vi "eGateHSP_Init.vi"(0 "e.gate Configuration":T1 {"StartTime" format="%#.10f"; "dActTimeToSecondFactor" format="%#.10f"; "StartTimeToDayFactor" format="%#_10f"}, 1 "DLL Path":path, 5 "IP-Adresse":string, 7 "mode":i32, 9 "sampleRate":i32, 11 "error in":errorcluster caption="Fehler (Eingang, kein Fehler)", 12 "timeout":i32) -> (4 "e.gate Configuration 2":T1 {"StartTime" format="%#.10f"; "dActTimeToSecondFactor" format="%#.10f"; "StartTimeToDayFactor" format="%#_10f"}, 15 "Fehler (Ausgang)":errorcluster)   [LabVIEW 2016]
uses:
  e.gate Configuration.ctl
  e.gate Channel Data.ctl
  e.gate Data Type.ctl
  e.gate Protocol Type.ctl
  e.gate Module  Data.ctl
  e.gateHSP_DLLhandle.ctl
panel:
  out "Rückgabewert":i32
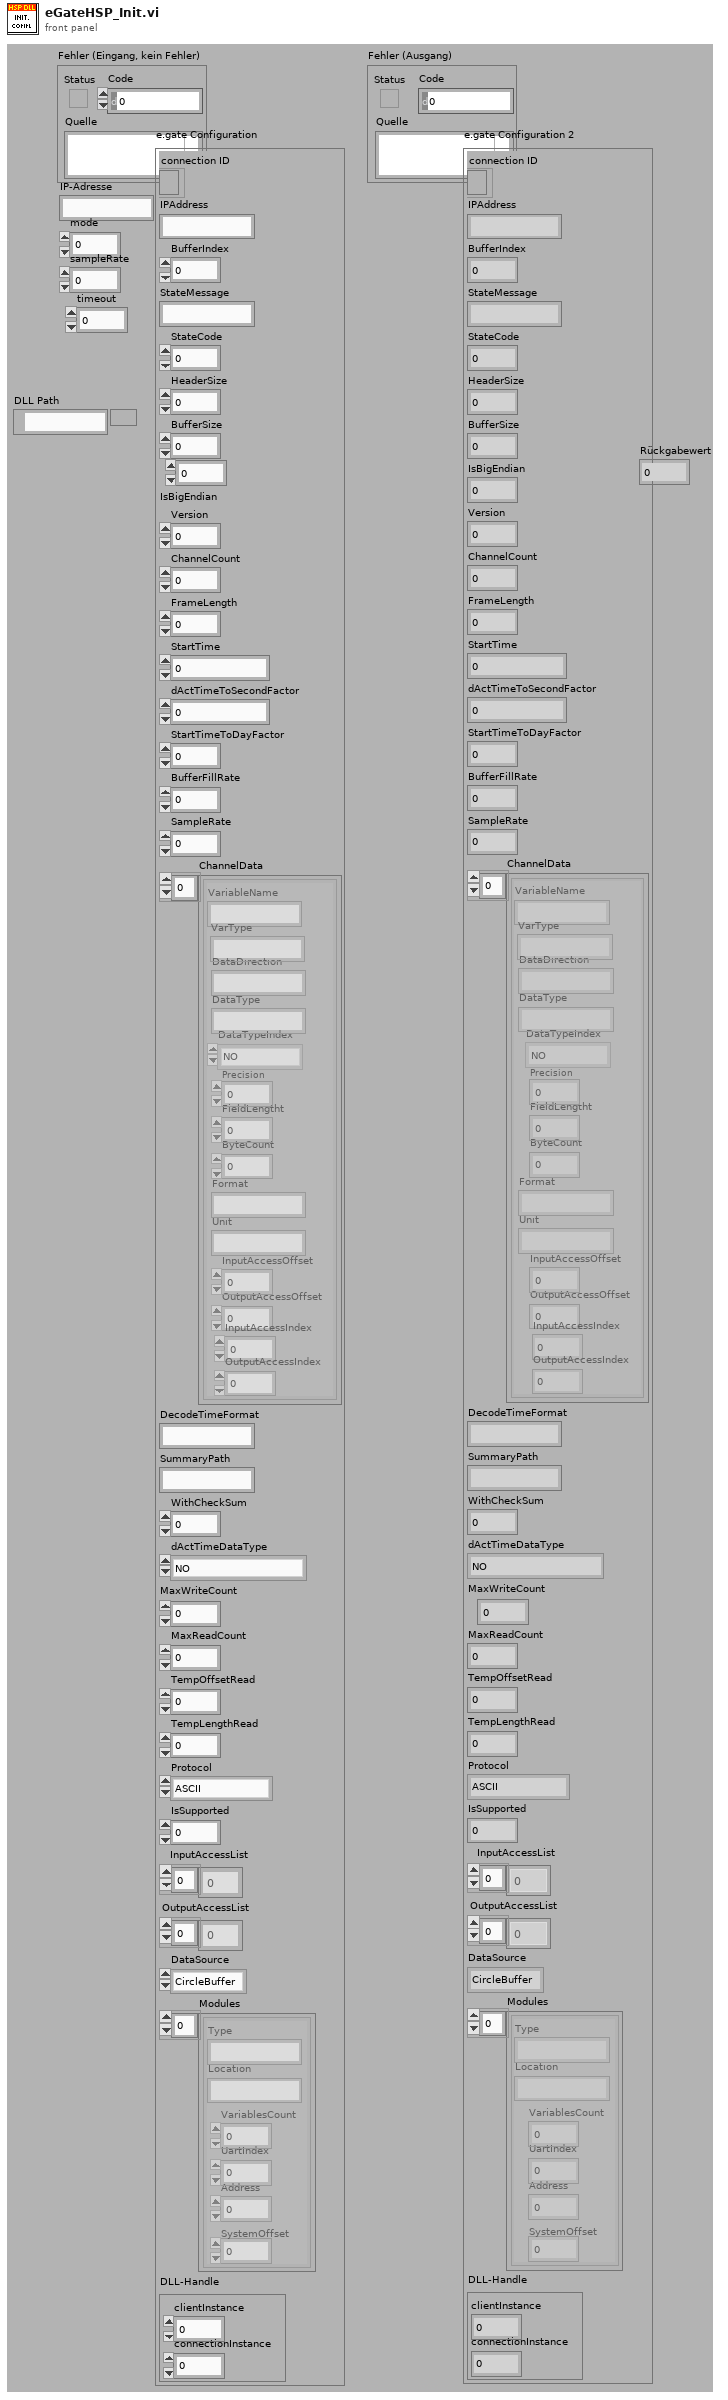
[diagram p1: front panel]
types:
  T1 = typedef "e.gate Configuration.ctl" = cluster{"connection ID":refnum<k5>, "IPAddress":string, "BufferIndex":i32, "StateMessage":string, "StateCode":i8, "HeaderSize":i32, "BufferSize":i32, "IsBigEndian":i32, "Version":i32, "ChannelCount":i32, "FrameLength":i32, "StartTime":dbl, "dActTimeToSecondFactor":dbl, "StartTimeToDayFactor":dbl, "BufferFillRate":dbl, "SampleRate":dbl, "ChannelData":T2[], "DecodeTimeFormat":string, "SummaryPath":string, "WithCheckSum":i32, "dActTimeDataType":T3, "MaxWriteCount":i32, "MaxReadCount":i32, "TempOffsetRead":i32, "TempLengthRead":i32, "Protocol":T4, "IsSupported":i32, "InputAccessList":i32[], "OutputAccessList":i32[], "DataSource":enum16{"CircleBuffer", "test.con Logger", "test.con Archive"}, "Modules":T5[], "DLL-Handle":T6}
  T2 = typedef "e.gate Channel Data.ctl" = cluster{"VariableName":string, "DataDirection":string, "DataType":string, "DataTypeIndex":T3, "Precision":i16, "FieldLengtht":i16, "ByteCount":i32, "Format":string, "Unit":string, "InputAccessOffset":i32, "OutputAccessOffset":i16, "InputAccessIndex":i16, "OutputAccessIndex":i16, "VarType":string}
  T3 = typedef "e.gate Data Type.ctl" = enum16{"NO", "BOOL", "SINT8", "USINT8", "SINT16", "USINT16", "SINT32", "USINT32", "FLOAT", "SET8", "SET16", "SET32", "DOUBLE", "SINT64", "USINT64", "SET64"}
  T4 = typedef "e.gate Protocol Type.ctl" = enum16{"ASCII", "HighspeedPort Online", "HighspeedPort Buffer", "eGateHighspeedPortDLL "}
  T5 = typedef "e.gate Module  Data.ctl" = cluster{"Type":string, "Location":string, "VariablesCount":i16, "UartIndex":i16, "Address":i16, "SystemOffset":i16}
  T6 = typedef "e.gateHSP_DLLhandle.ctl" = cluster{"clientInstance":i32, "connectionInstance":i32}
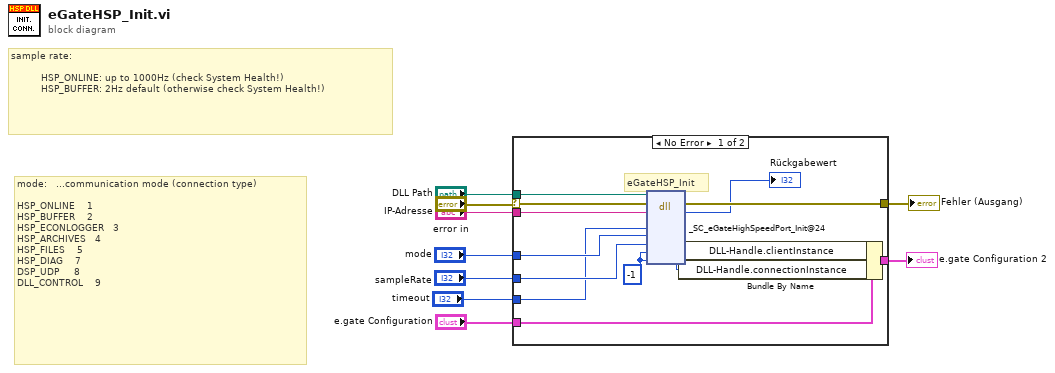
[diagram p0: block diagram]
diagram:
  # "sample rate:\n\n\t\t\t\t\t\t\t\t  HSP_ONLINE: up to 1000Hz (check System Health!)\n\t\t\t\t\t\t\t\t  HSP_BUFFER: 2Hz default (otherwise check System Health!)"
  # "mode:   ...communication mode (connection type)\n\nHSP_ONLINE\t\t\t\t1\nHSP_BUFFER\t\t\t\t2\nHSP_ECONLOGGER\t\t\t3\nHSP_ARCHIVES\t\t\t4\nHSP_FILES\t\t\t\t5\nHSP_DIAG\t\t\t\t7\nDSP_UDP\t\t\t\t\t8\nDLL_CONTROL\t\t\t\t9"
  n1 = case shown="No Error" "error in" {
    selector: "error in" -> [w21 w23]
    tunnel: [w17 w23] -> w8
    tunnel: "IP-Adresse" -> [w20 _]
    tunnel: "mode" -> [w19 _]
    tunnel: "sampleRate" -> [w18 _]
    tunnel: [w14 _] -> w3
    tunnel: "e.gate Configuration" -> [w15 _]
    tunnel: "timeout" -> [w16 _]
    tunnel: "DLL Path" -> [w10 _]
    frame No Error {
      w22 = -1 ("clientInstance")
      # "eGateHSP_Init"
      n2 = dll-call lib="PTH2abs E00. ç³»ç»éæ$17S007 11æ-Gantnerééå°-ç§¦é·SourceCodes0125HardWareGantner\nGantnerDriver\nGantnerDLLeGateHighSpeedPort.dll" fn="_SC_eGateHighSpeedPort_Init@24"(path in=w10, error in=w21, "hostName"=w20, "timeout"=w16, "mode"=w19, "sampleRate"=w18, "clientInstance"=w22, "connectionInstance"=w22) -> (error out=w17:errorcluster, "Rückgabewert"=→"Rückgabewert":i32, "clientInstance"=w13:i32, "connectionInstance"=w12:i32)  [unwired: 5 in, 1 out]
      n3 = Bundle By Name(cluster=w15, "DLL-Handle.clientInstance"=w13, "DLL-Handle.connectionInstance"=w12) -> (w14:T1)
    }
    frame Error {
    }
  }
  "Fehler (Ausgang)" <- w8
  "e.gate Configuration 2" <- w3
